vi "Omniax_mDrive_COM9_MM.vi"() -> ()   [LabVIEW 2009]
uses:
  <vilib>/Instr/_visa.llb/VISA Configure Serial Port (Instr).vi
panel:
  in  "Y Scan set":bool
  in  "Y Scan Velocity SP mm/sec":dbl
  in  "Y Scan Length SP mm":dbl
  in  "Y Move Set":bool
  out "Backlash steps/sec":i32
  out "Backlash":i32
  out "Y in Motion":bool
  in  "Reset":bool
  out "Reset Motor Step to":dbl
  in  "Reset Y Position to":dbl
  out "Y Velocity MV mm/sec":dbl
  in  "Y Velocity SP mm/sec":dbl
  in  "Y Position SP mm":dbl
  out "Y Position MV mm":dbl
  out "Holding Current %":i32
  out "Run Current %":i32
  out "Y Scan velocity MV mm/sec":dbl format="%#_6f"
  out "Y Scan length MV mm":dbl
  in  "Y Scan Cancel":bool
  out "Y Position mm PV":dbl
  out "offset":dbl
  out "mm/rev":dbl
  out "steps/rev":u32
  out "scan steps/secm return":i32
  in  "Y Scan Length SP steps":i32 min=-460800 max=460800 step=100
  out "Y Scan":bool
  in  "Y Scan Set":bool
  in  "Scan Go":bool
  in  "Y Velocity SP step/sec":i32
  in  "Y Scan Velocity SP steps/sec":i32=1 min=1 max=102400 step=1
  in  "Stop":bool
  out "Y in Range":bool
  out "Y Step PV":i32 max=2000
  out "Status":string
  in  "Go":bool
  in  "Y Step SP":i32=-20000 min=-460800 max=460800 step=500
  out "MINPOS":i32=-94296
  out "MAXPOS":i32=-34296
  out "COM PORT":refnum<visa-resource-name>="COM5"
  # "SY"
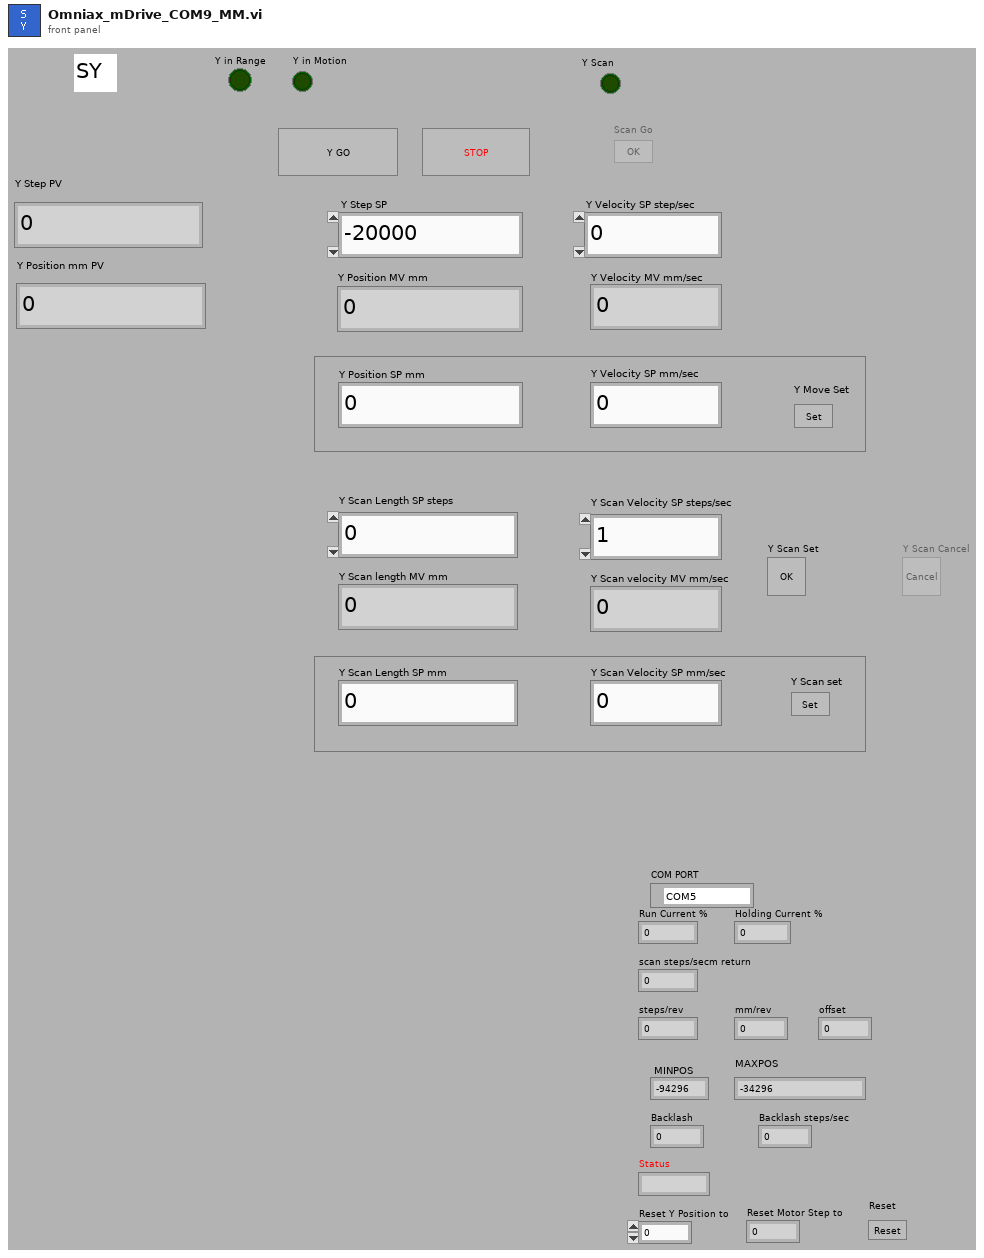
[diagram p1: front panel]
types:
  T1 = enum8{"Enabled", "Disabled", "Disabled and Grayed Out"}
  T2 = enum16{"Stop", "Reset", "Run Current", "Holding Current", "Accel Rate", "Decel Rate", "Move to Relative Position", "Move to Absolute Position", "Echo Mode", "Print Parameter", "Send String", "Microstep Resolution", "Set Current Position", "Max Velocity"}
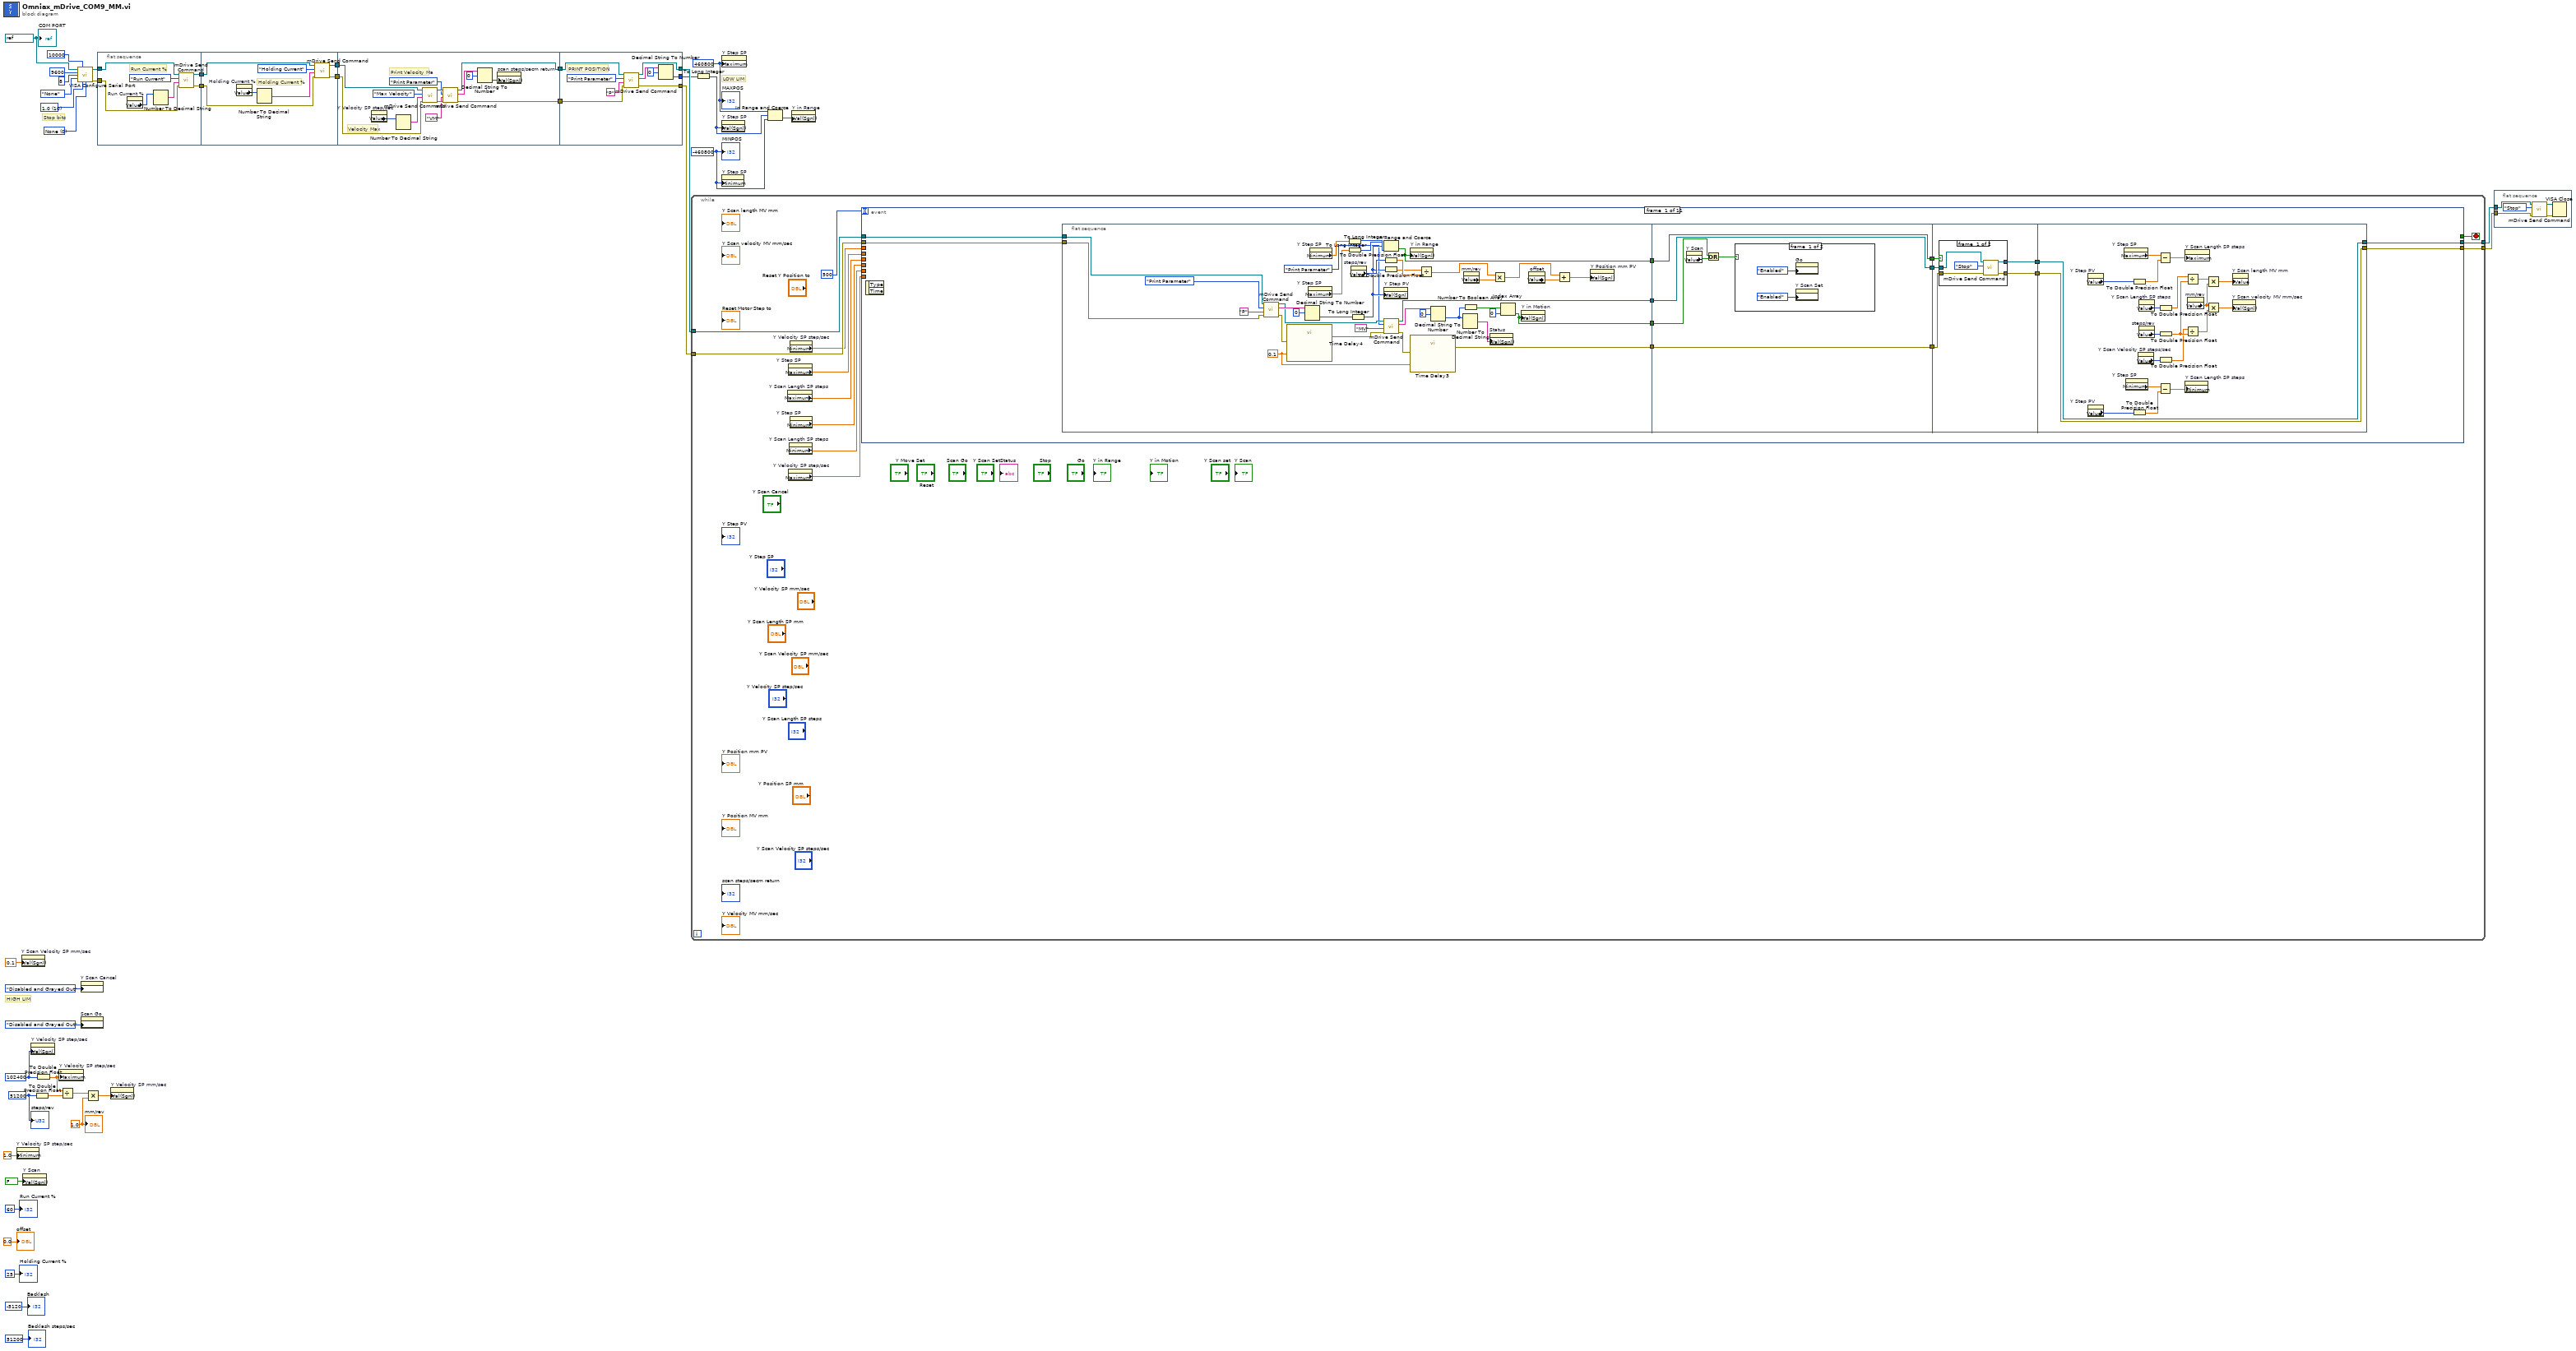
[diagram p0: block diagram]
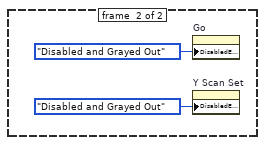
[diagram p2: hidden frame]
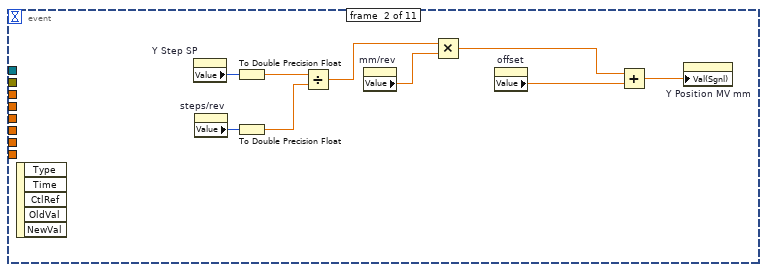
[diagram p4: hidden frame]
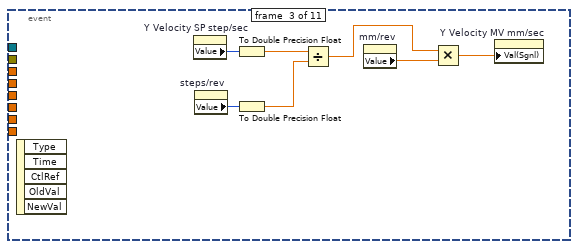
[diagram p5: hidden frame]
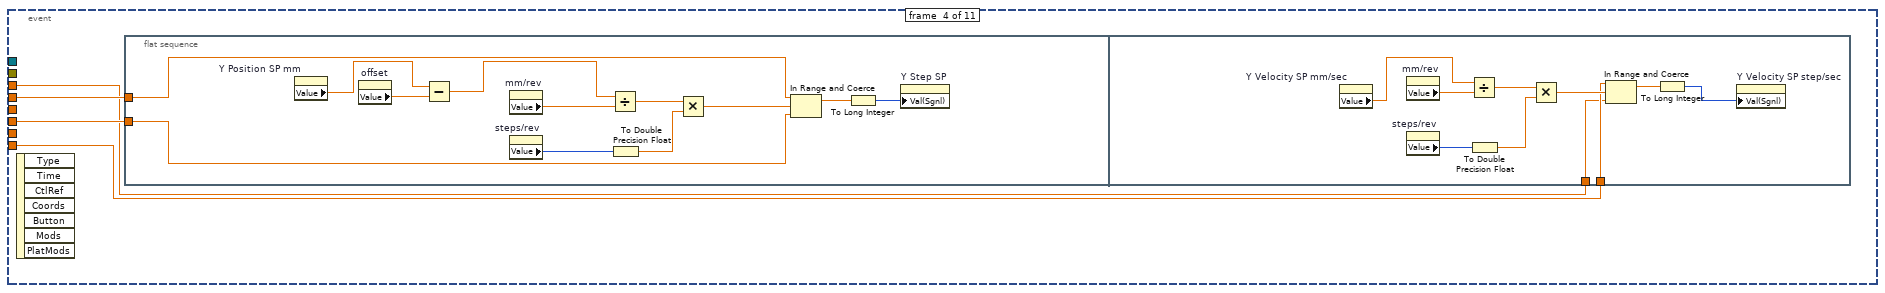
[diagram p6: hidden frame]
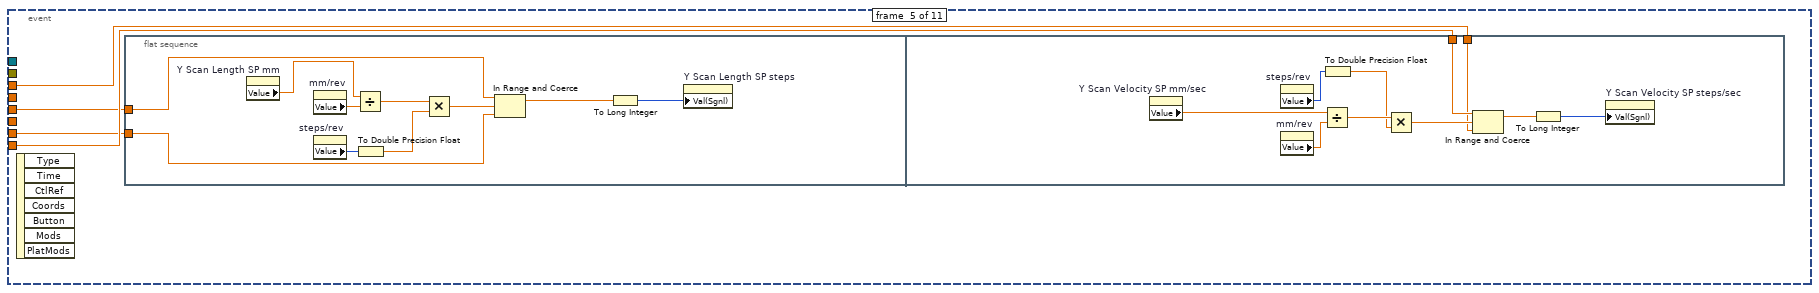
[diagram p7: hidden frame]
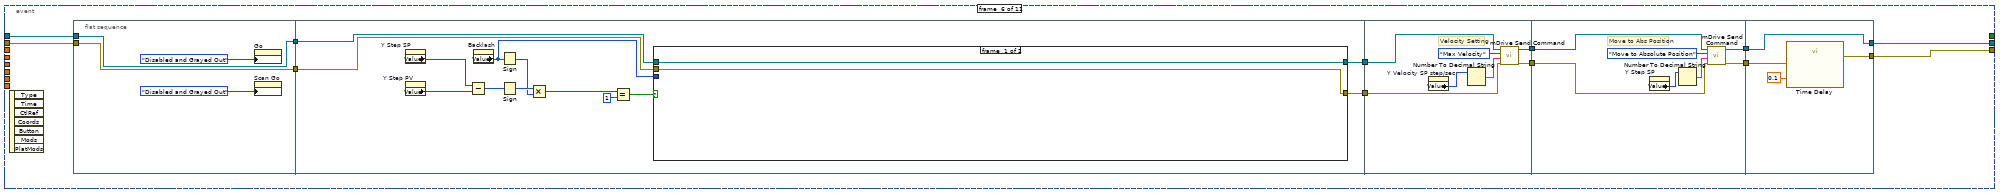
[diagram p8: hidden frame]
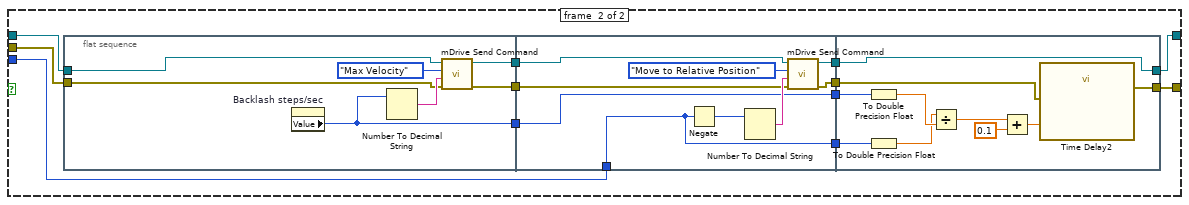
[diagram p9: hidden frame]
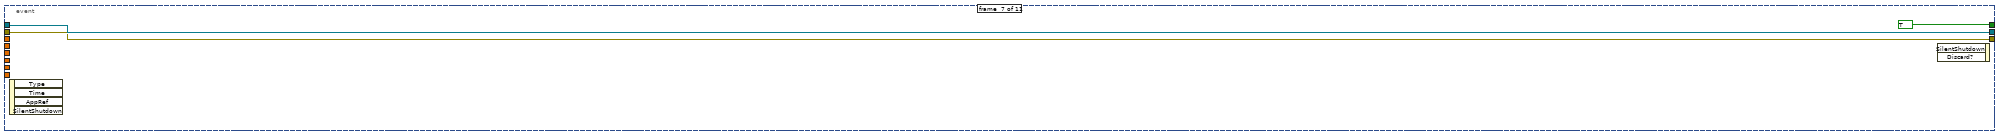
[diagram p10: hidden frame]
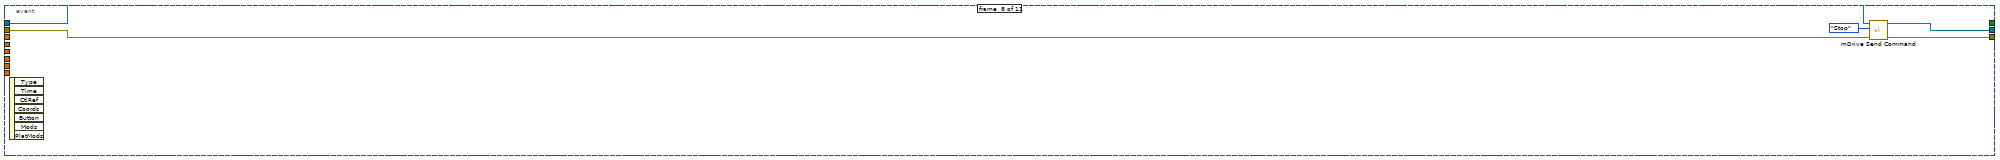
[diagram p11: hidden frame]
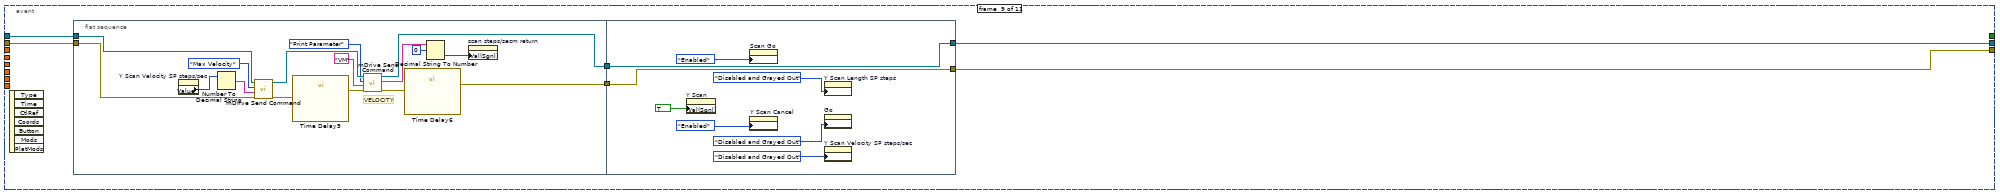
[diagram p12: hidden frame]
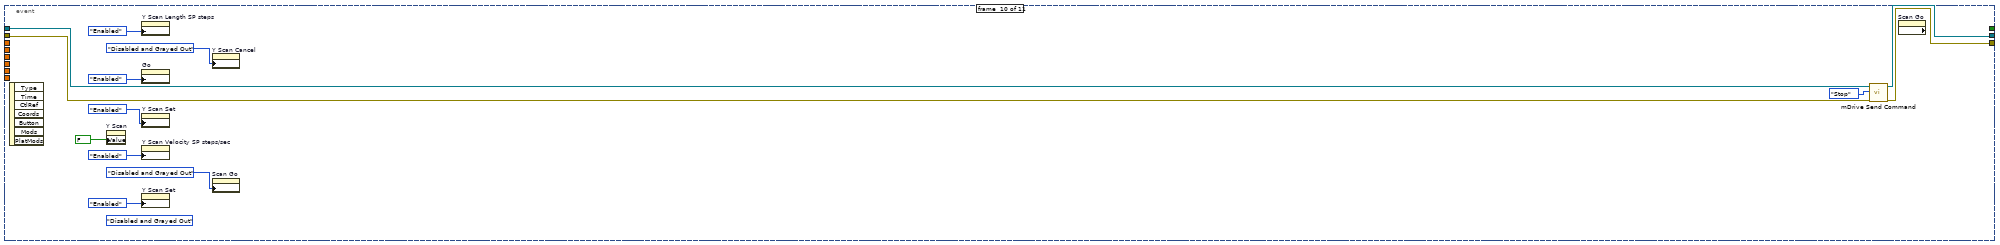
[diagram p13: hidden frame]
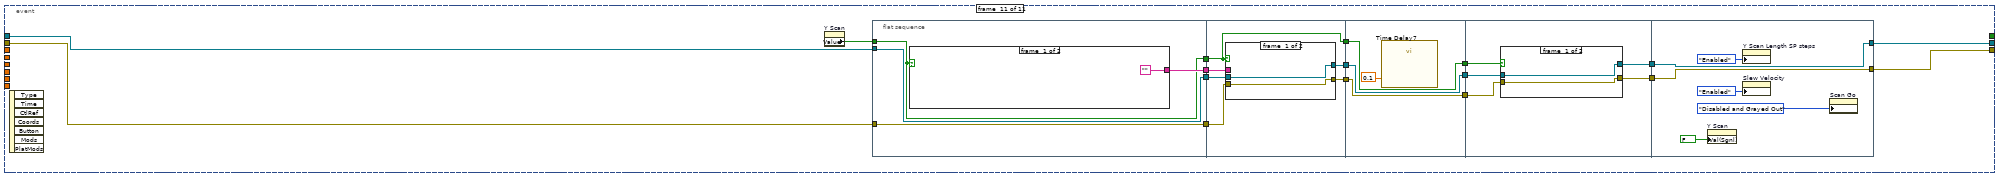
[diagram p14: hidden frame]
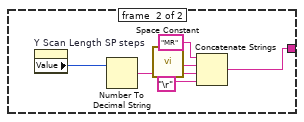
[diagram p15: hidden frame]
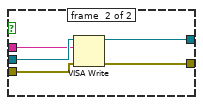
[diagram p16: hidden frame]
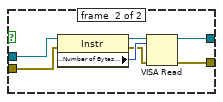
[diagram p17: hidden frame]
diagram:
  w6 = 1.0 ("MM/rev")
  w3 = u32 51200 ("step/rev")
  w8 = 102400 ("Value (Signaling)")
  w28 = -460800 ("lower limit")
  w27 = 460800 ("upper limit")
  w35 = refnum<visa-resource-name> "COM9" ("COM PORT")
  w37 = u16 0 items=["None", "XON/XOFF", "RTS/CTS", "XON/XOFF & RTS/CTS", "DTR/DSR", "XON/XOFF & DTR/DSR"] ("flow control (0:none)")
  w38 = u16 10 items=["1.0"=10, "1.5"=15, "2.0"=20] ("stop bits (10: 1 bit)")
  # "HIGH LIM"
  # "LOW LIM"
  # "Stop bits"
  n1 = property on="Y Velocity SP step/sec" class="DigNum (strict)"("Minimum"=1.0 ("Data Entry Limits:Minimum")) -> ()  [unwired: 2 in, 2 out]
  n2 = property on="Y Scan Velocity SP mm/sec" class="DigNum (strict)"("Val(Sgnl)"=0.1 ("Value (Signaling)")) -> ()  [unwired: 2 in, 2 out]
  n3 = property on="Y Scan" class="Bool (strict)"("Val(Sgnl)"=FALSE ("Value (Signaling)")) -> ()  [unwired: 2 in, 2 out]
  n4 = property on="Y Velocity SP step/sec" class="DigNum (strict)"("Val(Sgnl)"=w8) -> ()  [unwired: 2 in, 2 out]
  n5 = To Double Precision Float(number=w3) -> (double precision float=w4:dbl)
  n6 = To Double Precision Float(number=w8) -> (double precision float=w2:dbl)
  n7 = property on="Y Velocity SP step/sec" class="DigNum (strict)"("Maximum"=w2) -> ()  [unwired: 2 in, 2 out]
  n8 = Divide(x=w2, y=w4) -> (x/y=w7:dbl)
  n9 = call-poly "VISA Configure Serial Port"("VISA resource name"=w35, "timeout (10sec)"=u32 10000, "baud rate (9600)"=u32 9600, "data bits (8)"=u16 8, "parity (0:none)"=enum16{"None", "Odd", "Even", "Mark", "Space"}."None", "stop bits (10: 1 bit)"=w38, "flow control (0:none)"=w37) -> ("VISA resource name out"=w23:refnum<visa-resource-name>, "error out"=w22:errorcluster)  [unwired: 7 in]
  n10 = property on="Y Scan Cancel" class="Bool"("DisabledEnum"=T1."Disabled and Grayed Out" ("Disabled")) -> ()  [unwired: 2 in, 2 out]
  n11 = property on="Scan Go" class="Bool"("DisabledEnum"=T1."Disabled and Grayed Out" ("Disabled")) -> ()  [unwired: 2 in, 2 out]
  n12 = Multiply(x=w7, y=w6) -> (x*y=w5:dbl)
  n13 = flat-sequence {
    tunnel: w22 -> [w48]
    tunnel: w23 -> [w46]
    tunnel: [w45] -> w17
    tunnel: [w47] -> w15
    tunnel: w17 -> [w55]
    tunnel: [w54] -> w16
    tunnel: w15 -> [w52]
    tunnel: [w53] -> w14
    tunnel: [w65] -> w25
    tunnel: [w66] -> w24
    tunnel: w16 -> [w64]
    tunnel: w14 -> [w63]
    tunnel: [w78] -> w34
    tunnel: [w77] -> w33
    tunnel: [w72] -> w26
    tunnel: w25 -> [w76]
    tunnel: w24 -> [w75]
    frame #0 {
      # "Run Current %"
      n14 = property on="Run Current %" class="DigNum (strict)"() -> ("Value"=w43:i32)  [unwired: 2 in, 2 out]
      n15 = Number To Decimal String(number=w43) -> (decimal integer string=w44:string)  [unwired: 1 in]
      n16 = call "mDrive Send Command.vi"("error in (no error)"=w48, "Extra"=w44, "Command"=T2."Run Current", "VISA resource name"=w46) -> ("error out"=w47:errorcluster, "VISA resource name out"=w45:refnum<visa-resource-name>)  [unwired: 3 in, 1 out]
    }
    frame #1 {
      # "Holding Current %"
      n17 = property on="Holding Current %" class="DigNum (strict)"() -> ("Value"=w50:i32)  [unwired: 2 in, 2 out]
      n18 = Number To Decimal String(number=w50) -> (decimal integer string=w51:string)  [unwired: 1 in]
      n19 = call "mDrive Send Command.vi"("error in (no error)"=w52, "Extra"=w51, "Command"=T2."Holding Current", "VISA resource name"=w55) -> ("error out"=w53:errorcluster, "VISA resource name out"=w54:refnum<visa-resource-name>)  [unwired: 3 in, 1 out]
    }
    frame #2 {
      # "Print Velocity Ma"
      # "Velocity Max"
      n20 = property on="Y Velocity SP step/sec" class="DigNum (strict)"() -> ("Value"=w62:i32)  [unwired: 2 in, 2 out]
      n21 = Number To Decimal String(number=w62) -> (decimal integer string=w61:string)  [unwired: 1 in]
      n22 = call "mDrive Send Command.vi"("error in (no error)"=w63, "Extra"=w61, "Command"=T2."Max Velocity", "VISA resource name"=w64) -> ("error out"=w59:errorcluster, "VISA resource name out"=w69:refnum<visa-resource-name>)  [unwired: 3 in, 1 out]
      n23 = call "mDrive Send Command.vi"("error in (no error)"=w59, "Extra"="VM", "Command"=T2."Print Parameter", "VISA resource name"=w69) -> ("error out"=w66:errorcluster, "read buffer"=w67:string, "VISA resource name out"=w65:refnum<visa-resource-name>)  [unwired: 3 in]
      n24 = Decimal String To Number(string=w67, offset=0) -> (number=w60:i32)  [unwired: 1 in, 1 out]
      n25 = property on="scan steps/secm return" class="DigNum (strict)"("Val(Sgnl)"=w60) -> ()  [unwired: 2 in, 2 out]
    }
    frame #3 {
      # "PRINT POSITION"
      n26 = call "mDrive Send Command.vi"("error in (no error)"=w75, "Extra"="P", "Command"=T2."Print Parameter", "VISA resource name"=w76) -> ("error out"=w77:errorcluster, "read buffer"=w74:string, "VISA resource name out"=w78:refnum<visa-resource-name>)  [unwired: 3 in]
      n27 = Decimal String To Number(string=w74, offset=0) -> (number=w72:i32)  [unwired: 1 in, 1 out]
    }
  }
  n28 = property on="Y Velocity SP mm/sec" class="DigNum (strict)"("Val(Sgnl)"=w5) -> ()  [unwired: 2 in, 2 out]
  n29 = while {
    tunnel: w34 -> [w86]
    tunnel: w33 -> [w89]
    tunnel: [w90] -> w30
    tunnel: [w88] -> w31
    stop <- w85 stop-if-true
    n30 = property on="Y Scan Length SP steps" class="DigNum (strict)"() -> ("Maximum"=w79:dbl)  [unwired: 2 in, 2 out]
    n31 = property on="Y Step SP" class="DigNum (strict)"() -> ("Maximum"=w83:dbl)  [unwired: 2 in, 2 out]
    n32 = property on="Y Velocity SP step/sec" class="DigNum (strict)"() -> ("Maximum"=w82:dbl)  [unwired: 2 in, 2 out]
    n33 = property on="Y Scan Length SP steps" class="DigNum (strict)"() -> ("Minimum"=w80:dbl)  [unwired: 2 in, 2 out]
    n34 = property on="Y Velocity SP step/sec" class="DigNum (strict)"() -> ("Minimum"=w81:dbl)  [unwired: 2 in, 2 out]
    n35 = property on="Y Step SP" class="DigNum (strict)"() -> ("Minimum"=w84:dbl)  [unwired: 2 in, 2 out]
    n36 = event shown="[10] \"Scan Go\": Mouse Up" {
      selector: _ -> [_ _ _ _ _ _ _ _ _ _ _]
      dyn-events: _ -> [_ _ _ _ _ _ _ _ _ _ _]
      timeout: 500 -> [_ _ _ _ _ _ _ _ _ _ _]
      tunnel: w89 -> [w103 _ _ _ _ w254 w338 w343 w350 w380 w404]
      tunnel: [w102 _ _ _ _ w260 w338 w341 w348 w382 w401] -> w90
      tunnel: w86 -> [w100 _ _ _ _ w255 w339 w344 w349 w381 w403]
      tunnel: [w101 _ _ _ _ w261 w339 w342 w345 w383 w402] -> w88
      tunnel: [_ _ _ _ _ _ TRUE _ _ _ _] -> w85
      tunnel: w84 -> [_ _ _ w203 _ _ _ _ _ _ _]
      tunnel: w83 -> [_ _ _ w202 _ _ _ _ _ _ _]
      tunnel: w82 -> [_ _ _ w201 w229 _ _ _ _ _ _]
      tunnel: w81 -> [_ _ _ w200 w228 _ _ _ _ _ _]
      tunnel: w80 -> [_ _ _ _ w227 _ _ _ _ _ _]
      tunnel: w79 -> [_ _ _ _ w226 _ _ _ _ _ _]
      event #0 {
        n37 = event-data() -> ()  [unwired: 1 in, 2 out]
        n38 = flat-sequence {
          tunnel: w103 -> [w135]
          tunnel: w100 -> [w134]
          tunnel: [w140] -> w97
          tunnel: [w114] -> w95
          tunnel: [w127] -> w93
          tunnel: [w104] -> w91
          tunnel: w97 -> [w146]
          tunnel: [w146] -> w96
          tunnel: w95 -> [w145]
          tunnel: [w145] -> w94
          tunnel: w93 -> [w144]
          tunnel: [w144] -> w92
          tunnel: w91 -> [w143]
          tunnel: w96 -> [w152]
          tunnel: [w153] -> w99
          tunnel: w94 -> [w155]
          tunnel: [w154] -> w98
          tunnel: w92 -> [w151]
          tunnel: [w182] -> w102
          tunnel: [w183] -> w101
          tunnel: w99 -> [w183]
          tunnel: w98 -> [w182]
          frame #0 {
            w108 = 0.1 ("Delay Time (s)")
            n39 = call "mDrive Send Command.vi"("error in (no error)"=w135, "Extra"="P", "Command"=T2."Print Parameter", "VISA resource name"=w134) -> ("error out"=w133:errorcluster, "read buffer"=w139:string, "VISA resource name out"=w137:refnum<visa-resource-name>)  [unwired: 3 in]
            n40 = call "Time Delay4"("error in (no error)"=w133, "Delay Time (s)"=w108) -> ("error out"=w132:errorcluster)  [unwired: 9 in]
            n41 = Decimal String To Number(string=w139, offset=0) -> (number=w117:i32)  [unwired: 1 in, 1 out]
            n42 = property on="Y Step SP" class="DigNum (strict)"() -> ("Maximum"=w129:dbl)  [unwired: 2 in, 2 out]
            n43 = property on="Y Step SP" class="DigNum (strict)"() -> ("Minimum"=w131:dbl)  [unwired: 2 in, 2 out]
            n44 = To Long Integer(number=w131) -> (32bit integer=w130:i32)
            n45 = To Long Integer(number=w129) -> (32bit integer=w128:i32)
            n46 = To Long Integer(number=w117) -> (32bit integer=w119:i32)
            n47 = property on="steps/rev" class="DigNum (strict)"() -> ("Value"=w125:u32)  [unwired: 2 in, 2 out]
            n48 = In Range and Coerce(upper limit=w128, x=w119, lower limit=w130) -> (In Range?=w127:bool)  [unwired: 1 out]
            n49 = To Double Precision Float(number=w125) -> (double precision float=w126:dbl)
            n50 = To Double Precision Float(number=w119) -> (double precision float=w120:dbl)
            n51 = property on="Y Step PV" class="DigNum (strict)"("Val(Sgnl)"=w119) -> ()  [unwired: 2 in, 2 out]
            n52 = call "mDrive Send Command.vi"("error in (no error)"=w132, "Extra"="MV", "Command"=T2."Print Parameter", "VISA resource name"=w137) -> ("error out"=w136:errorcluster, "read buffer"=w115:string, "VISA resource name out"=w140:refnum<visa-resource-name>)  [unwired: 3 in]
            n53 = property on="Y in Range" class="Bool (strict)"("Val(Sgnl)"=w127) -> ()  [unwired: 2 in, 2 out]
            n54 = call "Time Delay3"("error in (no error)"=w136, "Delay Time (s)"=w108) -> ("error out"=w114:errorcluster)  [unwired: 9 in]
            n55 = Divide(x=w120, y=w126) -> (x/y=w124:dbl)
            n56 = Decimal String To Number(string=w115, offset=0 ("offset (0)")) -> (number=w107:i32)  [unwired: 1 in, 1 out]
            n57 = Number To Decimal String(number=w107) -> (decimal integer string=w113:string)  [unwired: 1 in]
            n58 = property on="mm/rev" class="DigNum (strict)"() -> ("Value"=w123:dbl)  [unwired: 2 in, 2 out]
            n59 = Number To Boolean Array(number=w107) -> (Boolean array=w106:bool[])
            n60 = property on="Status" class="Str"("Val(Sgnl)"=w113) -> ()  [unwired: 2 in, 2 out]
            n61 = Multiply(x=w124, y=w123) -> (x*y=w122:dbl)
            n62 = Index Array(array=w106, index=0) -> (element=w104:bool)
            n63 = property on="Y in Motion" class="Bool (strict)"("Val(Sgnl)"=w104) -> ()  [unwired: 2 in, 2 out]
            n64 = property on="offset" class="DigNum (strict)"() -> ("Value"=w121:dbl)  [unwired: 2 in, 2 out]
            n65 = Add(x=w122, y=w121) -> (x+y=w118:dbl)
            n66 = property on="Y Position mm PV" class="DigNum (strict)"("Val(Sgnl)"=w118) -> ()  [unwired: 2 in, 2 out]
          }
          frame #1 {
            n67 = property on="Y Scan" class="Bool (strict)"() -> ("Value"=w141:bool)  [unwired: 2 in, 2 out]
            n68 = Or(x=w143, y=w141) -> (x .or. y?=w142:bool)
            n69 = case shown="False" w142 {
              frame #0 {
                n70 = property on="Go" class="Bool"("DisabledEnum"=T1."Enabled" ("Disabled")) -> ()  [unwired: 2 in, 2 out]
                n71 = property on="Y Scan Set" class="Bool"("DisabledEnum"=T1."Enabled" ("Disabled")) -> ()  [unwired: 2 in, 2 out]
              }
              frame #1 {
                n72 = property on="Go" class="Bool"("DisabledEnum"=T1."Disabled and Grayed Out" ("Disabled")) -> ()  [unwired: 2 in, 2 out]
                n73 = property on="Y Scan Set" class="Bool"("DisabledEnum"=T1."Disabled and Grayed Out" ("Disabled")) -> ()  [unwired: 2 in, 2 out]
              }
            }
          }
          frame #2 {
            n74 = case shown="False" w151 {
              tunnel: w152 -> [w158 w162]
              tunnel: [w159 w162] -> w153
              tunnel: [w160 w161] -> w154
              tunnel: w155 -> [w157 w161]
              frame #0 {
                n75 = call "mDrive Send Command.vi"("error in (no error)"=w157, "Command"=T2."Stop", "VISA resource name"=w158) -> ("error out"=w160:errorcluster, "VISA resource name out"=w159:refnum<visa-resource-name>)  [unwired: 4 in, 1 out]
              }
              frame #1 {
              }
            }
          }
          frame #3 {
            n76 = property on="Y Step PV" class="DigNum (strict)"() -> ("Value"=w172:i32)  [unwired: 2 in, 2 out]
            n77 = property on="Y Step PV" class="DigNum (strict)"() -> ("Value"=w170:i32)  [unwired: 2 in, 2 out]
            n78 = property on="Y Step SP" class="DigNum (strict)"() -> ("Maximum"=w179:dbl)  [unwired: 2 in, 2 out]
            n79 = property on="Y Step SP" class="DigNum (strict)"() -> ("Minimum"=w180:dbl)  [unwired: 2 in, 2 out]
            n80 = To Double Precision Float(number=w172) -> (double precision float=w171:dbl)
            n81 = To Double Precision Float(number=w170) -> (double precision float=w169:dbl)
            n82 = property on="Y Scan Velocity SP steps/sec" class="DigNum (strict)"() -> ("Value"=w167:i32)  [unwired: 2 in, 2 out]
            n83 = property on="Y Scan Length SP steps" class="DigNum (strict)"() -> ("Value"=w176:i32)  [unwired: 2 in, 2 out]
            n84 = property on="steps/rev" class="DigNum (strict)"() -> ("Value"=w174:u32)  [unwired: 2 in, 2 out]
            n85 = Subtract(x=w179, y=w171) -> (x-y=w178:dbl)
            n86 = Subtract(x=w180, y=w169) -> (x-y=w181:dbl)
            n87 = To Double Precision Float(number=w176) -> (double precision float=w175:dbl)
            n88 = To Double Precision Float(number=w174) -> (double precision float=w168:dbl)
            n89 = To Double Precision Float(number=w167) -> (double precision float=w166:dbl)
            n90 = property on="Y Scan Length SP steps" class="DigNum (strict)"("Maximum"=w178) -> ()  [unwired: 2 in, 2 out]
            n91 = Divide(x=w175, y=w168) -> (x/y=w177:dbl)
            n92 = Divide(x=w166, y=w168) -> (x/y=w165:dbl)
            n93 = property on="Y Scan Length SP steps" class="DigNum (strict)"("Minimum"=w181) -> ()  [unwired: 2 in, 2 out]
            n94 = property on="mm/rev" class="DigNum (strict)"() -> ("Value"=w173:dbl)  [unwired: 2 in, 2 out]
            n95 = Multiply(x=w177, y=w173) -> (x*y=w164:dbl)
            n96 = Multiply(x=w173, y=w165) -> (x*y=w163:dbl)
            n97 = property on="Y Scan length MV mm" class="DigNum (strict)"("Value"=w164) -> ()  [unwired: 2 in, 2 out]
            n98 = property on="Y Scan velocity MV mm/sec" class="DigNum (strict)"("Val(Sgnl)"=w163) -> ()  [unwired: 2 in, 2 out]
          }
        }
      }
      event #1 {
        n99 = event-data() -> ()  [unwired: 1 in, 5 out]
        n100 = property on="Y Step SP" class="DigNum (strict)"() -> ("Value"=w185:i32)  [unwired: 2 in, 2 out]
        n101 = property on="steps/rev" class="DigNum (strict)"() -> ("Value"=w186:u32)  [unwired: 2 in, 2 out]
        n102 = To Double Precision Float(number=w185) -> (double precision float=w187:dbl)
        n103 = To Double Precision Float(number=w186) -> (double precision float=w192:dbl)
        n104 = Divide(x=w187, y=w192) -> (x/y=w191:dbl)
        n105 = property on="mm/rev" class="DigNum (strict)"() -> ("Value"=w190:dbl)  [unwired: 2 in, 2 out]
        n106 = Multiply(x=w191, y=w190) -> (x*y=w189:dbl)
        n107 = property on="offset" class="DigNum (strict)"() -> ("Value"=w188:dbl)  [unwired: 2 in, 2 out]
        n108 = Add(x=w189, y=w188) -> (x+y=w184:dbl)
        n109 = property on="Y Position MV mm" class="DigNum (strict)"("Val(Sgnl)"=w184) -> ()  [unwired: 2 in, 2 out]
      }
      event #2 {
        n110 = event-data() -> ()  [unwired: 1 in, 5 out]
        n111 = property on="Y Velocity SP step/sec" class="DigNum (strict)"() -> ("Value"=w194:i32)  [unwired: 2 in, 2 out]
        n112 = property on="steps/rev" class="DigNum (strict)"() -> ("Value"=w195:u32)  [unwired: 2 in, 2 out]
        n113 = To Double Precision Float(number=w194) -> (double precision float=w196:dbl)
        n114 = To Double Precision Float(number=w195) -> (double precision float=w199:dbl)
        n115 = Divide(x=w196, y=w199) -> (x/y=w198:dbl)
        n116 = property on="mm/rev" class="DigNum (strict)"() -> ("Value"=w197:dbl)  [unwired: 2 in, 2 out]
        n117 = Multiply(x=w198, y=w197) -> (x*y=w193:dbl)
        n118 = property on="Y Velocity MV mm/sec" class="DigNum (strict)"("Val(Sgnl)"=w193) -> ()  [unwired: 2 in, 2 out]
      }
      event #3 {
        n119 = event-data() -> ()  [unwired: 1 in, 7 out]
        n120 = flat-sequence {
          tunnel: w203 -> [w206]
          tunnel: w202 -> [w205]
          tunnel: w201 -> [w218]
          tunnel: w200 -> [w217]
          frame #0 {
            n121 = property on="Y Position SP mm" class="DigNum (strict)"() -> ("Value"=w208:dbl)  [unwired: 2 in, 2 out]
            n122 = property on="offset" class="DigNum (strict)"() -> ("Value"=w209:dbl)  [unwired: 2 in, 2 out]
            n123 = Subtract(x=w208, y=w209) -> (x-y=w213:dbl)
            n124 = property on="mm/rev" class="DigNum (strict)"() -> ("Value"=w212:dbl)  [unwired: 2 in, 2 out]
            n125 = property on="steps/rev" class="DigNum (strict)"() -> ("Value"=w211:u32)  [unwired: 2 in, 2 out]
            n126 = Divide(x=w213, y=w212) -> (x/y=w214:dbl)
            n127 = To Double Precision Float(number=w211) -> (double precision float=w215:dbl)
            n128 = Multiply(x=w214, y=w215) -> (x*y=w207:dbl)
            n129 = In Range and Coerce(upper limit=w205, x=w207, lower limit=w206) -> (coerced(x)=w204:dbl)  [unwired: 1 out]
            n130 = To Long Integer(number=w204) -> (32bit integer=w210:i32)
            n131 = property on="Y Step SP" class="DigNum (strict)"("Val(Sgnl)"=w210) -> ()  [unwired: 2 in, 2 out]
          }
          frame #1 {
            n132 = property on="Y Velocity SP mm/sec" class="DigNum (strict)"() -> ("Value"=w223:dbl)  [unwired: 2 in, 2 out]
            n133 = property on="mm/rev" class="DigNum (strict)"() -> ("Value"=w225:dbl)  [unwired: 2 in, 2 out]
            n134 = property on="steps/rev" class="DigNum (strict)"() -> ("Value"=w221:u32)  [unwired: 2 in, 2 out]
            n135 = Divide(x=w223, y=w225) -> (x/y=w224:dbl)
            n136 = To Double Precision Float(number=w221) -> (double precision float=w222:dbl)
            n137 = Multiply(x=w224, y=w222) -> (x*y=w219:dbl)
            n138 = In Range and Coerce(upper limit=w218, x=w219, lower limit=w217) -> (coerced(x)=w216:dbl)  [unwired: 1 out]
            n139 = To Long Integer(number=w216) -> (32bit integer=w220:i32)
            n140 = property on="Y Velocity SP step/sec" class="DigNum (strict)"("Val(Sgnl)"=w220) -> ()  [unwired: 2 in, 2 out]
          }
        }
      }
      event #4 {
        n141 = event-data() -> ()  [unwired: 1 in, 7 out]
        n142 = flat-sequence {
          tunnel: w227 -> [w231]
          tunnel: w226 -> [w230]
          tunnel: w229 -> [w241]
          tunnel: w228 -> [w240]
          frame #0 {
            n143 = property on="Y Scan Length SP mm" class="DigNum (strict)"() -> ("Value"=w234:dbl)  [unwired: 2 in, 2 out]
            n144 = property on="mm/rev" class="DigNum (strict)"() -> ("Value"=w237:dbl)  [unwired: 2 in, 2 out]
            n145 = property on="steps/rev" class="DigNum (strict)"() -> ("Value"=w236:u32)  [unwired: 2 in, 2 out]
            n146 = Divide(x=w234, y=w237) -> (x/y=w238:dbl)
            n147 = To Double Precision Float(number=w236) -> (double precision float=w239:dbl)
            n148 = Multiply(x=w238, y=w239) -> (x*y=w233:dbl)
            n149 = In Range and Coerce(upper limit=w230, x=w233, lower limit=w231) -> (coerced(x)=w232:dbl)  [unwired: 1 out]
            n150 = To Long Integer(number=w232) -> (32bit integer=w235:i32)
            n151 = property on="Y Scan Length SP steps" class="DigNum (strict)"("Val(Sgnl)"=w235) -> ()  [unwired: 2 in, 2 out]
          }
          frame #1 {
            n152 = property on="Y Scan Velocity SP mm/sec" class="DigNum (strict)"() -> ("Value"=w247:dbl)  [unwired: 2 in, 2 out]
            n153 = property on="steps/rev" class="DigNum (strict)"() -> ("Value"=w245:u32)  [unwired: 2 in, 2 out]
            n154 = property on="mm/rev" class="DigNum (strict)"() -> ("Value"=w249:dbl)  [unwired: 2 in, 2 out]
            n155 = Divide(x=w247, y=w249) -> (x/y=w248:dbl)
            n156 = To Double Precision Float(number=w245) -> (double precision float=w246:dbl)
            n157 = Multiply(x=w248, y=w246) -> (x*y=w243:dbl)
            n158 = In Range and Coerce(upper limit=w241, x=w243, lower limit=w240) -> (coerced(x)=w242:dbl)  [unwired: 1 out]
            n159 = To Long Integer(number=w242) -> (32bit integer=w244:i32)
            n160 = property on="Y Scan Velocity SP steps/sec" class="DigNum (strict)"("Val(Sgnl)"=w244) -> ()  [unwired: 2 in, 2 out]
          }
        }
      }
      event #5 {
        n161 = event-data() -> ()  [unwired: 1 in, 7 out]
        n162 = flat-sequence {
          tunnel: w254 -> [w264]
          tunnel: w255 -> [w265]
          tunnel: [w265] -> w251
          tunnel: [w264] -> w250
          tunnel: [w267] -> w253
          tunnel: [w266] -> w252
          tunnel: w251 -> [w269]
          tunnel: w250 -> [w268]
          tunnel: [w322] -> w257
          tunnel: [w321] -> w256
          tunnel: w253 -> [w320]
          tunnel: w252 -> [w319]
          tunnel: [w329] -> w259
          tunnel: [w328] -> w258
          tunnel: w257 -> [w327]
          tunnel: w256 -> [w326]
          tunnel: [w335] -> w260
          tunnel: [w336] -> w261
          tunnel: w259 -> [w336]
          tunnel: w258 -> [w334]
          frame #0 {
            n163 = property on="Go" class="Bool"("DisabledEnum"=T1."Disabled and Grayed Out" ("Disabled")) -> ()  [unwired: 2 in, 2 out]
            n164 = property on="Scan Go" class="Bool"("DisabledEnum"=T1."Disabled and Grayed Out" ("Disabled")) -> ()  [unwired: 2 in, 2 out]
          }
          frame #1 {
            n165 = property on="Y Step SP" class="DigNum (strict)"() -> ("Value"=w278:i32)  [unwired: 2 in, 2 out]
            n166 = property on="Y Step PV" class="DigNum (strict)"() -> ("Value"=w277:i32)  [unwired: 2 in, 2 out]
            n167 = Subtract(x=w278, y=w277) -> (x-y=w276:i32)
            n168 = property on="Backlash" class="DigNum (strict)"() -> ("Value"=w270:i32)  [unwired: 2 in, 2 out]
            n169 = Sign(1:w270) -> (0:w274:i32)
            n170 = Sign(1:w276) -> (0:w275:i32)
            n171 = Multiply(x=w275, y=w274) -> (x*y=w273:i32)
            n172 = Equal?(x=w273, y=1) -> (x = y?=w271:bool)
            n173 = case shown="True" w271 {
              tunnel: w270 -> [_ w289]
              tunnel: w269 -> [w280 w292]
              tunnel: w268 -> [w279 w291]
              tunnel: [w279 w283] -> w267
              tunnel: [w280 w281] -> w266
              frame #0 {
              }
              frame #1 {
                n174 = flat-sequence {
                  tunnel: w292 -> [w297]
                  tunnel: w291 -> [w296]
                  tunnel: [w293] -> w290
                  tunnel: [w295] -> w286
                  tunnel: [w294] -> w285
                  tunnel: w290 -> [w306]
                  tunnel: w289 -> [w300]
                  tunnel: [w306] -> w288
                  tunnel: [w300] -> w287
                  tunnel: w286 -> [w305]
                  tunnel: w285 -> [w304]
                  tunnel: [w303] -> w284
                  tunnel: [w302] -> w282
                  tunnel: w288 -> [w315]
                  tunnel: w287 -> [w314]
                  tunnel: w284 -> [w311]
                  tunnel: [w310] -> w283
                  tunnel: [w309] -> w281
                  tunnel: w282 -> [w309]
                  frame #0 {
                    n175 = property on="Backlash steps/sec" class="DigNum (strict)"() -> ("Value"=w293:i32)  [unwired: 2 in, 2 out]
                    n176 = Number To Decimal String(number=w293) -> (decimal integer string=w298:string)  [unwired: 1 in]
                    n177 = call "mDrive Send Command.vi"("error in (no error)"=w296, "Extra"=w298, "Command"=T2."Max Velocity", "VISA resource name"=w297) -> ("error out"=w294:errorcluster, "VISA resource name out"=w295:refnum<visa-resource-name>)  [unwired: 3 in, 1 out]
                  }
                  frame #1 {
                    n178 = Negate(x=w300) -> (-x=w301:i32)
                    n179 = Number To Decimal String(number=w301) -> (decimal integer string=w307:string)  [unwired: 1 in]
                    n180 = call "mDrive Send Command.vi"("error in (no error)"=w304, "Extra"=w307, "Command"=T2."Move to Relative Position", "VISA resource name"=w305) -> ("error out"=w303:errorcluster, "VISA resource name out"=w302:refnum<visa-resource-name>)  [unwired: 3 in, 1 out]
                  }
                  frame #2 {
                    n181 = To Double Precision Float(number=w315) -> (double precision float=w317:dbl)
                    n182 = To Double Precision Float(number=w314) -> (double precision float=w313:dbl)
                    n183 = Divide(x=w313, y=w317) -> (x/y=w318:dbl)
                    n184 = Add(x=w318, y=0.1) -> (x+y=w312:dbl)
                    n185 = call "Time Delay2"("error in (no error)"=w311, "Delay Time (s)"=w312) -> ("error out"=w310:errorcluster)  [unwired: 9 in]
                  }
                }
              }
            }
          }
          frame #2 {
            # "Velocity Setting"
            n186 = property on="Y Velocity SP step/sec" class="DigNum (strict)"() -> ("Value"=w323:i32)  [unwired: 2 in, 2 out]
            n187 = Number To Decimal String(number=w323) -> (decimal integer string=w324:string)  [unwired: 1 in]
            n188 = call "mDrive Send Command.vi"("error in (no error)"=w320, "Extra"=w324, "Command"=T2."Max Velocity", "VISA resource name"=w319) -> ("error out"=w321:errorcluster, "VISA resource name out"=w322:refnum<visa-resource-name>)  [unwired: 3 in, 1 out]
          }
          frame #3 {
            # "Move to Abs Position"
            n189 = property on="Y Step SP" class="DigNum (strict)"() -> ("Value"=w332:i32)  [unwired: 2 in, 2 out]
            n190 = Number To Decimal String(number=w332) -> (decimal integer string=w331:string)  [unwired: 1 in]
            n191 = call "mDrive Send Command.vi"("error in (no error)"=w326, "Extra"=w331, "Command"=T2."Move to Absolute Position", "VISA resource name"=w327) -> ("error out"=w328:errorcluster, "VISA resource name out"=w329:refnum<visa-resource-name>)  [unwired: 3 in, 1 out]
          }
          frame #4 {
            n192 = call "Time Delay"("error in (no error)"=w334, "Delay Time (s)"=0.1) -> ("error out"=w335:errorcluster)  [unwired: 9 in]
          }
        }
      }
      event #6 {
        n193 = event-data() -> ()  [unwired: 1 in, 4 out]
        n194 = event-data() -> ()  [unwired: 3 in, 1 out]
      }
      event #7 {
        n195 = event-data() -> ()  [unwired: 1 in, 7 out]
        n196 = call "mDrive Send Command.vi"("error in (no error)"=w343, "Command"=T2."Stop", "VISA resource name"=w344) -> ("error out"=w341:errorcluster, "VISA resource name out"=w342:refnum<visa-resource-name>)  [unwired: 4 in, 1 out]
      }
      event #8 {
        n197 = event-data() -> ()  [unwired: 1 in, 7 out]
        n198 = flat-sequence {
          tunnel: w350 -> [w360]
          tunnel: w349 -> [w359]
          tunnel: [w356] -> w347
          tunnel: [w354] -> w346
          tunnel: [w373] -> w348
          tunnel: [w374] -> w345
          tunnel: w347 -> [w374]
          tunnel: w346 -> [w373]
          frame #0 {
            # "VELOCITY"
            n199 = property on="Y Scan Velocity SP steps/sec" class="DigNum (strict)"() -> ("Value"=w357:i32)  [unwired: 2 in, 2 out]
            n200 = Number To Decimal String(number=w357) -> (decimal integer string=w358:string)  [unwired: 1 in]
            n201 = call "mDrive Send Command.vi"("error in (no error)"=w360, "Extra"=w358, "Command"=T2."Max Velocity", "VISA resource name"=w359) -> ("error out"=w361:errorcluster, "VISA resource name out"=w366:refnum<visa-resource-name>)  [unwired: 3 in, 1 out]
            n202 = call "Time Delay5"("error in (no error)"=w361) -> ("error out"=w364:errorcluster)  [unwired: 10 in]
            n203 = call "mDrive Send Command.vi"("error in (no error)"=w364, "Extra"="VM", "Command"=T2."Print Parameter", "VISA resource name"=w366) -> ("error out"=w355:errorcluster, "read buffer"=w362:string, "VISA resource name out"=w356:refnum<visa-resource-name>)  [unwired: 3 in]
            n204 = call "Time Delay6"("error in (no error)"=w355) -> ("error out"=w354:errorcluster)  [unwired: 10 in]
            n205 = Decimal String To Number(string=w362, offset=0) -> (number=w365:i32)  [unwired: 1 in, 1 out]
            n206 = property on="scan steps/secm return" class="DigNum (strict)"("Val(Sgnl)"=w365) -> ()  [unwired: 2 in, 2 out]
          }
          frame #1 {
            n207 = property on="Y Scan" class="Bool (strict)"("Val(Sgnl)"=TRUE ("Slew Ready 2")) -> ()  [unwired: 2 in, 2 out]
            n208 = property on="Scan Go" class="Bool"("DisabledEnum"=T1."Enabled" ("Disabled")) -> ()  [unwired: 2 in, 2 out]
            n209 = property on="Y Scan Cancel" class="Bool"("DisabledEnum"=T1."Enabled" ("Disabled")) -> ()  [unwired: 2 in, 2 out]
            n210 = property on="Y Scan Length SP steps" class="DigNum (strict)"("DisabledEnum"=T1."Disabled and Grayed Out" ("Disabled")) -> ()  [unwired: 2 in, 2 out]
            n211 = property on="Go" class="Bool"("DisabledEnum"=T1."Disabled and Grayed Out" ("Disabled")) -> ()  [unwired: 2 in, 2 out]
            n212 = property on="Y Scan Velocity SP steps/sec" class="DigNum (strict)"("DisabledEnum"=T1."Disabled and Grayed Out" ("Disabled")) -> ()  [unwired: 2 in, 2 out]
          }
        }
      }
      event #9 {
        (unwired) T1."Disabled and Grayed Out" ("Disabled")
        n213 = event-data() -> ()  [unwired: 1 in, 7 out]
        n214 = property on="Y Scan" class="Bool (strict)"("Value"=FALSE ("Slew Ready")) -> ()  [unwired: 2 in, 2 out]
        n215 = property on="Y Scan Length SP steps" class="DigNum (strict)"("DisabledEnum"=T1."Enabled" ("Disabled")) -> ()  [unwired: 2 in, 2 out]
        n216 = property on="Go" class="Bool"("DisabledEnum"=T1."Enabled" ("Disabled")) -> ()  [unwired: 2 in, 2 out]
        n217 = property on="Y Scan Set" class="Bool"("DisabledEnum"=T1."Enabled" ("Disabled")) -> ()  [unwired: 2 in, 2 out]
        n218 = property on="Y Scan Velocity SP steps/sec" class="DigNum (strict)"("DisabledEnum"=T1."Enabled" ("Disabled")) -> ()  [unwired: 2 in, 2 out]
        n219 = property on="Y Scan Set" class="Bool"("DisabledEnum"=T1."Enabled" ("Disabled")) -> ()  [unwired: 2 in, 2 out]
        n220 = property on="Y Scan Cancel" class="Bool"("DisabledEnum"=T1."Disabled and Grayed Out" ("Disabled")) -> ()  [unwired: 2 in, 2 out]
        n221 = property on="Scan Go" class="Bool"("DisabledEnum"=T1."Disabled and Grayed Out" ("Disabled")) -> ()  [unwired: 2 in, 2 out]
        n222 = call "mDrive Send Command.vi"("error in (no error)"=w380, "Command"=T2."Stop", "VISA resource name"=w381) -> ("error out"=w382:errorcluster, "VISA resource name out"=w383:refnum<visa-resource-name>)  [unwired: 4 in, 1 out]
        n223 = property on="Scan Go" class="Bool" props=["DisabledEnum"]() -> ()  [unwired: 2 in, 3 out]
      }
      event #10 {
        n224 = event-data() -> ()  [unwired: 1 in, 7 out]
        n225 = property on="Y Scan" class="Bool (strict)"() -> ("Value"=w391:bool)  [unwired: 2 in, 2 out]
        n226 = flat-sequence {
          tunnel: w404 -> [w407]
          tunnel: w403 -> [w408]
          tunnel: [w408] -> w400
          tunnel: [w407] -> w399
          tunnel: [w406] -> w398
          tunnel: w391 -> [w405]
          tunnel: [w405] -> w390
          tunnel: w400 -> [w419]
          tunnel: [w421] -> w395
          tunnel: w399 -> [w418]
          tunnel: [w420] -> w393
          tunnel: w398 -> [w417]
          tunnel: w390 -> [w416]
          tunnel: [w416] -> w388
          tunnel: w395 -> [w432]
          tunnel: [w432] -> w394
          tunnel: w393 -> [w431]
          tunnel: [w431] -> w392
          tunnel: [w429] -> w389
          tunnel: w388 -> [w429]
          tunnel: w394 -> [w437]
          tunnel: [w435] -> w397
          tunnel: w392 -> [w436]
          tunnel: [w434] -> w396
          tunnel: w389 -> [w433]
          tunnel: w397 -> [w452]
          tunnel: w396 -> [w451]
          tunnel: [w452] -> w402
          tunnel: [w451] -> w401
          frame #0 {
            n227 = case shown="True" w405 {
              tunnel: ["" w410] -> w406
              frame #0 {
              }
              frame #1 {
                n228 = property on="Y Scan Length SP steps" class="DigNum (strict)"() -> ("Value"=w415:i32)  [unwired: 2 in, 2 out]
                n229 = Number To Decimal String(number=w415) -> (decimal integer string=w412:string)  [unwired: 1 in]
                n230 = call <vilib>:"Space Constant.vi"() -> ("String"=w413:string)
                n231 = Concatenate Strings("MR", w413, w412, "\r") -> (w410:string)
              }
            }
          }
          frame #1 {
            n232 = case shown="True" w416 {
              tunnel: [w423 w428] -> w421
              tunnel: [w422 w427] -> w420
              tunnel: w419 -> [w423 w426]
              tunnel: w418 -> [w422 w425]
              tunnel: w417 -> [_ w424]
              frame #0 {
              }
              frame #1 {
                n233 = VISA Write(VISA resource name=w426, write buffer=w424, error in (no error)=w425) -> (VISA resource name out=w428:refnum<visa-resource-name>, error out=w427:errorcluster)  [unwired: 1 out]
              }
            }
          }
          frame #2 {
            n234 = call "Time Delay7"("Delay Time (s)"=0.1) -> ()  [unwired: 10 in, 1 out]
          }
          frame #3 {
            n235 = case shown="True" w433 {
              tunnel: w437 -> [w439 w443]
              tunnel: w436 -> [w438 w442]
              tunnel: [w439 w441] -> w435
              tunnel: [w438 w440] -> w434
              frame #0 {
              }
              frame #1 {
                n236 = property class="Instr"(reference=w443, error in=w442) -> (reference out=w445:refnum<visa-resource-name>, error out=w444:errorcluster, "Serial Settings:Number of Bytes at Serial Port"=w446:u32)
                n237 = VISA Read(VISA resource name=w445, byte count=w446, error in (no error)=w444) -> (VISA resource name out=w441:refnum<visa-resource-name>, error out=w440:errorcluster)  [unwired: 2 out]
              }
            }
          }
          frame #4 {
            n238 = property on="Y Scan" class="Bool (strict)"("Val(Sgnl)"=FALSE ("Slew Ready 2")) -> ()  [unwired: 2 in, 2 out]
            n239 = property on="Y Scan Length SP steps" class="DigNum (strict)"("DisabledEnum"=T1."Enabled" ("Disabled")) -> ()  [unwired: 2 in, 2 out]
            n240 = property on="Slew Velocity" class="DigNum (strict)"("DisabledEnum"=T1."Enabled" ("Disabled")) -> ()  [unwired: 2 in, 2 out]
            n241 = property on="Scan Go" class="Bool"("DisabledEnum"=T1."Disabled and Grayed Out" ("Disabled")) -> ()  [unwired: 2 in, 2 out]
          }
        }
      }
    }
  }
  n242 = To Long Integer(number=w26) -> (32bit integer=w32:i32)
  n243 = property on="Y Step SP" class="DigNum (strict)"("Maximum"=w27) -> ()  [unwired: 2 in, 2 out]
  n244 = property on="Y Step SP" class="DigNum (strict)"("Val(Sgnl)"=w32) -> ()  [unwired: 2 in, 2 out]
  n245 = property on="Y Step SP" class="DigNum (strict)"("Minimum"=w28) -> ()  [unwired: 2 in, 2 out]
  n246 = In Range and Coerce(upper limit=w27, x=w32, lower limit=w28) -> (In Range?=w29:bool)  [unwired: 1 out]
  n247 = property on="Y in Range" class="Bool (strict)"("Val(Sgnl)"=w29) -> ()  [unwired: 2 in, 2 out]
  n248 = flat-sequence {
    tunnel: w31 -> [w457]
    tunnel: w30 -> [w454]
    frame #0 {
      n249 = call "mDrive Send Command.vi"("error in (no error)"=w454, "Command"=T2."Stop", "VISA resource name"=w457) -> ("error out"=w455:errorcluster, "VISA resource name out"=w456:refnum<visa-resource-name>)  [unwired: 4 in, 1 out]
      n250 = VISA Close(VISA resource name=w456, error in (no error)=w455) -> ()  [unwired: 1 out]
    }
  }
  "COM PORT" <- w35
  "MINPOS" <- w28
  "MAXPOS" <- w27
  "steps/rev" <- w3
  "mm/rev" <- w6
  "offset" <- 0.0 ("offset")
  "Run Current %" <- 60 ("Run Current %")
  "Holding Current %" <- 25 ("Holding Current %")
  "Backlash" <- -5120 ("Backlash2")
  "Backlash steps/sec" <- 51200 ("Value (Signaling)")
